vi "Update Value by Index.vi"(4 "Raw":bool, 6 "Timestamp (Now)":dbl, 8 "error in (no error)":errorcluster, 9 "Scaled":bool, 10 "Index":i32, 11 "Group BOOL in":refnum<class "Group BOOL.lvclass">) -> (0 "error out":errorcluster, 3 "Group BOOL out":refnum<class "Group BOOL.lvclass">)   [LabVIEW 2020, in "Vecto.lvlib" / "Group BOOL.lvclass"]
uses:
  Group BOOL.lvclass
  Group BOOL.lvclass/Group BOOL.ctl
  Group/Group.lvclass
  C:/dev/lv20CE/relink/lv-vecto/Vecto/Group/Group.lvclass
  C:/dev/lv20CE/relink/lv-vecto/Vecto/Group BOOL/Group BOOL.lvclass
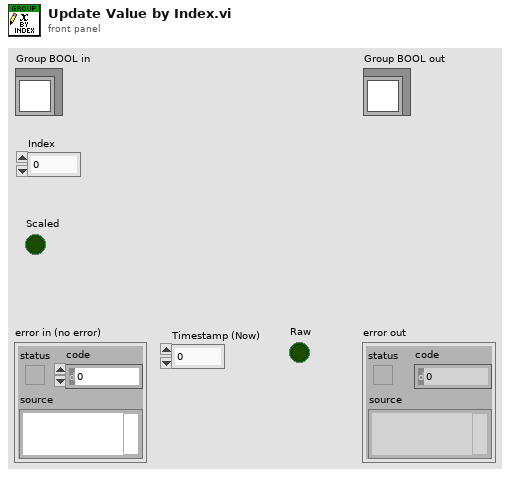
[diagram p1: front panel]
types:
  T1 = typedef "Vecto.lvlib/Group BOOL.lvclass/Ref.ctl" = cluster{"Scaled":bool[], "Timestamp":dbl[], "Raw":bool[]}
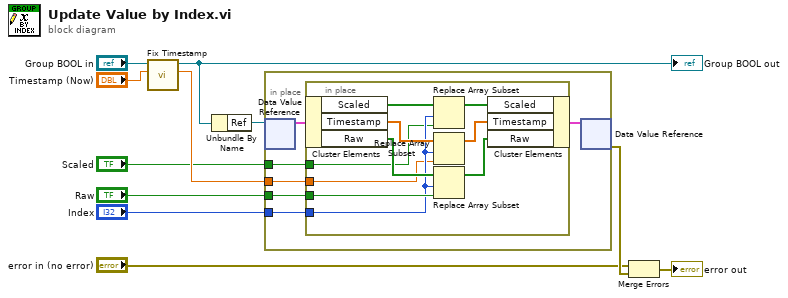
[diagram p0: block diagram]
diagram:
  n1 = call "Fix Timestamp.vi"("Timestamp in"="Timestamp (Now)", "GroupAbstract in"="Group BOOL in") -> ("Timestamp"=w9:dbl, "GroupAbstract out"=w7:refnum<class "Group BOOL.lvclass">)  [unwired: 7 in, 1 out]
  "Group BOOL out" <- w7
  n2 = Unbundle By Name(w7) -> ("Ref"=w11:refnum<data-value>)
  n3 = in-place {
    in-place-border: "Scaled" -> [w16]
    in-place-border: w9 -> [w15]
    in-place-border: "Raw" -> [w14]
    in-place-border: "Index" -> [w13]
    n4 = in-place-dvr #1(w11) -> (w17:T1)  [unwired: 1 out]
    n5 = in-place {
      in-place-border: w16 -> [w21]
      in-place-border: w15 -> [w22]
      in-place-border: w14 -> [w25]
      in-place-border: w13 -> [w23]
      n6 = in-place-cluster #2(w17) -> ("Scaled"=w27:bool[], "Timestamp"=w24:dbl[], "Raw"=w26:bool[])
      n7 = Replace Array Subset(array=w27, new element=w21, index=w23) -> (w20:bool[])
      n8 = Replace Array Subset(array=w24, new element=w22, index=w23) -> (w19:dbl[])
      n9 = Replace Array Subset(array=w26, new element=w25, index=w23) -> (w18:bool[])
      n10 = in-place-cluster #2("Scaled"=w20, "Timestamp"=w19, "Raw"=w18) -> (w12:T1)
    }
    n11 = in-place-dvr #1(w12) -> (w10:errorcluster)  [unwired: 1 out]
  }
  n12 = Merge Errors("error in (no error)", w10) -> (→"error out":errorcluster)
